vi "BooleanNotifier Send.vi"(8 "error in (no error)":errorcluster, 10 "boolean in":bool, 11 "BooleanNotifier in":refnum<class "BooleanNotifier.lvclass">) -> (0 "error out":errorcluster, 3 "BooleanNotifier out":refnum<class "BooleanNotifier.lvclass">)   [LabVIEW 2018, in "BooleanNotifier.lvclass"]
uses:
  BooleanNotifier.lvclass
  BooleanNotifier.lvclass/BooleanNotifier.ctl
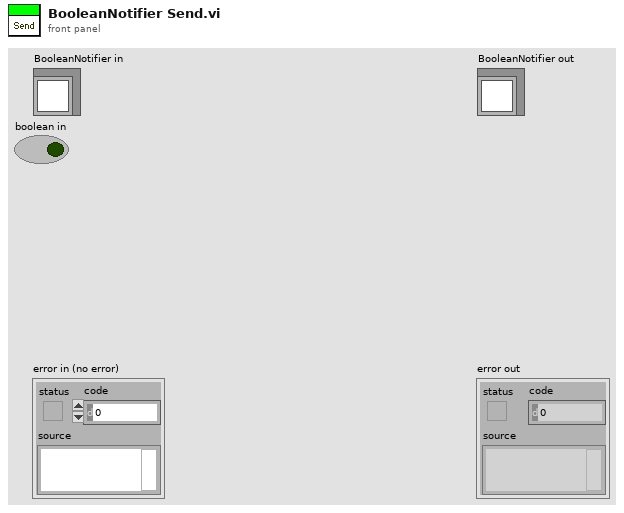
[diagram p1: front panel]
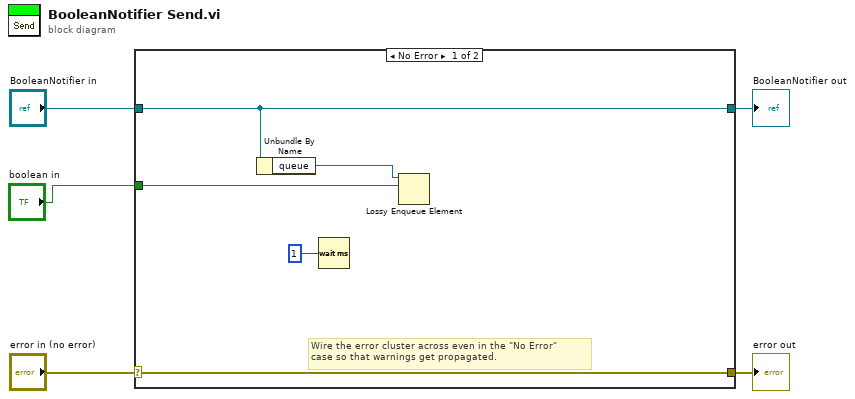
[diagram p0: block diagram]
diagram:
  n1 = case shown="No Error" "error in (no error)" {
    selector: "error in (no error)" -> [w10 w12]
    tunnel: [w10 w12] -> w4
    tunnel: [w9 w11] -> w2
    tunnel: "BooleanNotifier in" -> [w9 w11]
    tunnel: "boolean in" -> [w7 _]
    frame No Error {
      # "Wire the error cluster across even in the \"No Error\"\ncase so that warnings get propagated."
      n2 = Unbundle By Name(w9) -> ("queue"=w8:refnum<queue>)
      n3 = Wait (ms)(milliseconds to wait=u32 1) -> ()  [unwired: 1 out]
      n4 = Lossy Enqueue Element(queue=w8, element=w7) -> ()  [unwired: 1 in, 4 out]
    }
    frame Error {
    }
  }
  "error out" <- w4
  "BooleanNotifier out" <- w2
